vi "convertps-to-mmSD.vi"(1 "ps":dbl) -> (0 "mm":dbl)   [LabVIEW 2015]
uses:
  globalVarSD.vi
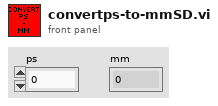
[diagram p1: front panel]
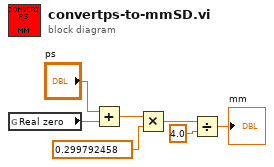
[diagram p0: block diagram]
diagram:
  n1 = global read "globalVarSD.vi" "Real zero"() -> (w1:dbl)
  n2 = Add(x="ps", y=w1) -> (x+y=w2:dbl)
  n3 = Multiply(x=w2, y=0.299792458) -> (x*y=w6:dbl)
  n4 = Divide(x=w6, y=4.0) -> (x/y=→"mm":dbl)
